vi "QPSK Demodulation.vi"(9 "pulse shaping filter (none)":T2(ring)) -> (0 "QPSK synchronization parameters":T3, 1 "matched filter coefficients":dbl[](array[numeric]), 3 "output bit stream":i8[](array[numeric]))   [LabVIEW 2026]
panel:
  out "PSK system parameters":T1 {"PSK type" items=["normal", "shifted", "offset"]; "symbol map" format="%.3f"}
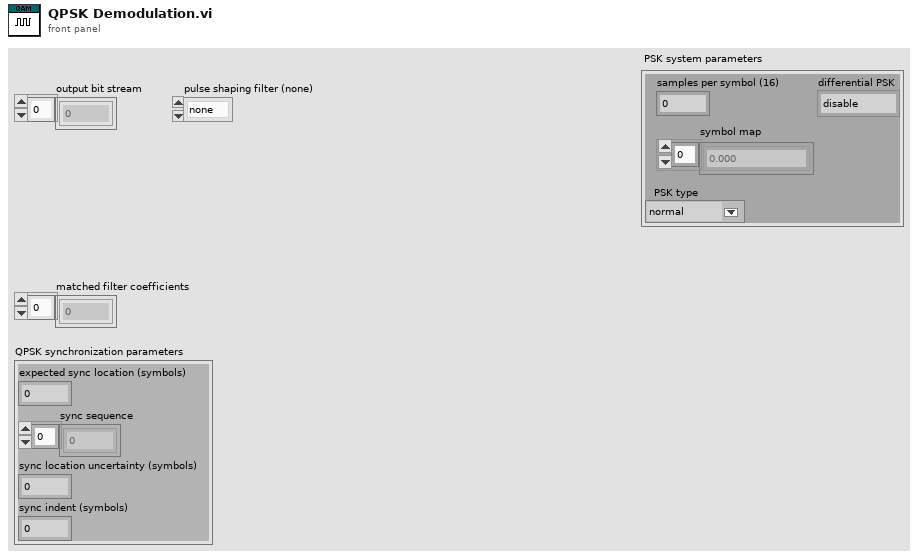
[diagram p1: front panel]
types:
  T1 = cluster{"samples per symbol (16)":i32, "symbol map":cdb[], "differential PSK":enum16{"disable", "enable"}, "PSK type":u16}
  T2 = enum16{"none", "Raised Cosine", "Root Raised Cos", "Gaussian"}
  T3 = cluster{"expected sync location (symbols)":i32, "sync sequence":cdb[], "sync location uncertainty (symbols)":i32, "sync indent (symbols)":i32}
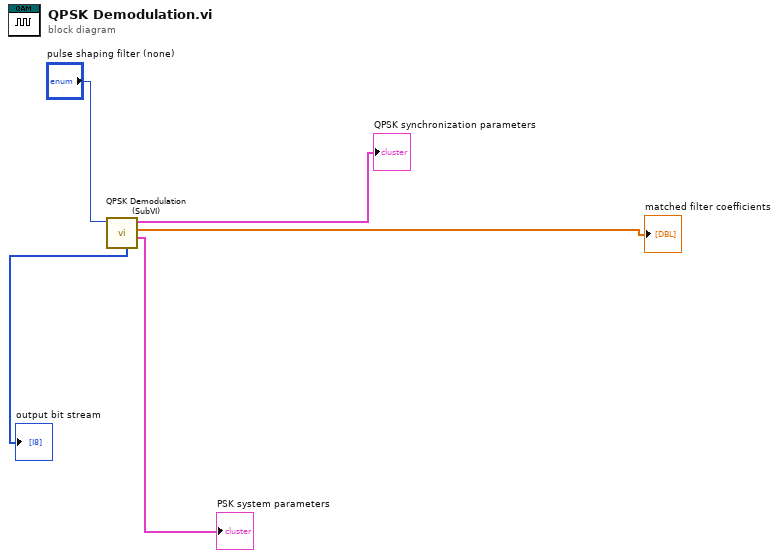
[diagram p0: block diagram]
diagram:
  n1 = call "QPSK Demodulation (SubVI).vi"("pulse shaping filter (none)"="pulse shaping filter (none)") -> ("PSK system parameters"=→"PSK system parameters":T1, "matched filter coefficients"=→"matched filter coefficients":dbl[], "QPSK synchronization parameters"=→"QPSK synchronization parameters":T3, "output bit stream"=→"output bit stream":i8[])  [unwired: 7 in]
